vi "sensor_msg.vi"(10 "motor_msg in":string, 11 "voltage_msg in":string) -> (3 "sensor_msg_cluster":cluster{"voltage":dbl, "motor":i8})   [LabVIEW 2014]
uses:
  <vilib>/Tufts CEEO ROS for LabVIEW Software/ROS/MessageParsing/std_msgs/subs/parse_float64_scalar.vi
  <vilib>/Tufts CEEO ROS for LabVIEW Software/ROS/MessageParsing/std_msgs/subs/parse_i8_scalar.vi
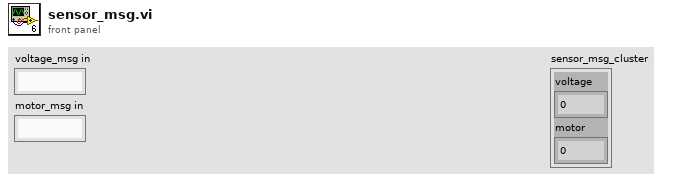
[diagram p1: front panel]
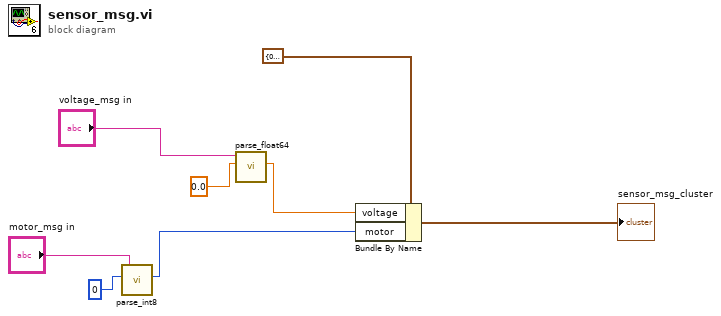
[diagram p0: block diagram]
diagram:
  n1 = call-poly <vilib>:"parse_int8.vi"("type"=i8 0, "msg in"="motor_msg in") -> ("number"=w3:i8)  [unwired: 3 in, 2 out]
  n2 = call-poly <vilib>:"parse_float64.vi"("type"=0.0, "msg in"="voltage_msg in") -> ("number"=w8:dbl)  [unwired: 3 in, 2 out]
  n3 = Bundle By Name(cluster=cluster{"voltage":dbl, "motor":i8} {"voltage"=0.0, "motor"=0} ("sensor"), "voltage"=w8, "motor"=w3) -> (→"sensor_msg_cluster":cluster{"voltage":dbl, "motor":i8})
